vi "SET LPF1.vi"(0 "NMR in":refnum<class "NMR.lvclass">, 5 "CuttOff Freq [MHz]":u8=9 min=1 max=30 step=1, 11 "error in (no error)":errorcluster) -> (4 "NMR out":refnum<class "NMR.lvclass">, 10 "String as ASCII":string, 15 "error out":errorcluster)   [LabVIEW 2011, in "NMR.lvclass"]
uses:
  NMR.lvclass
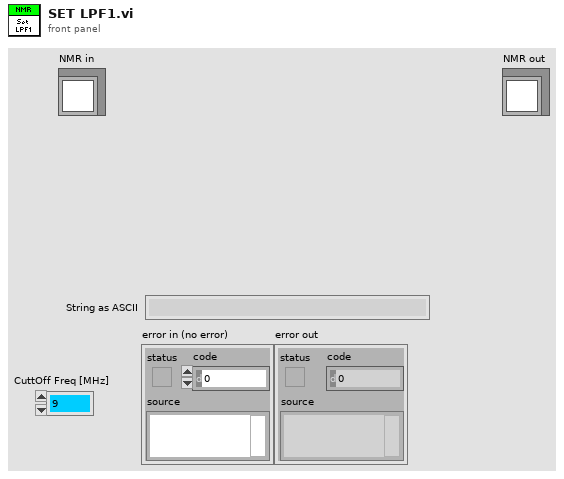
[diagram p1: front panel]
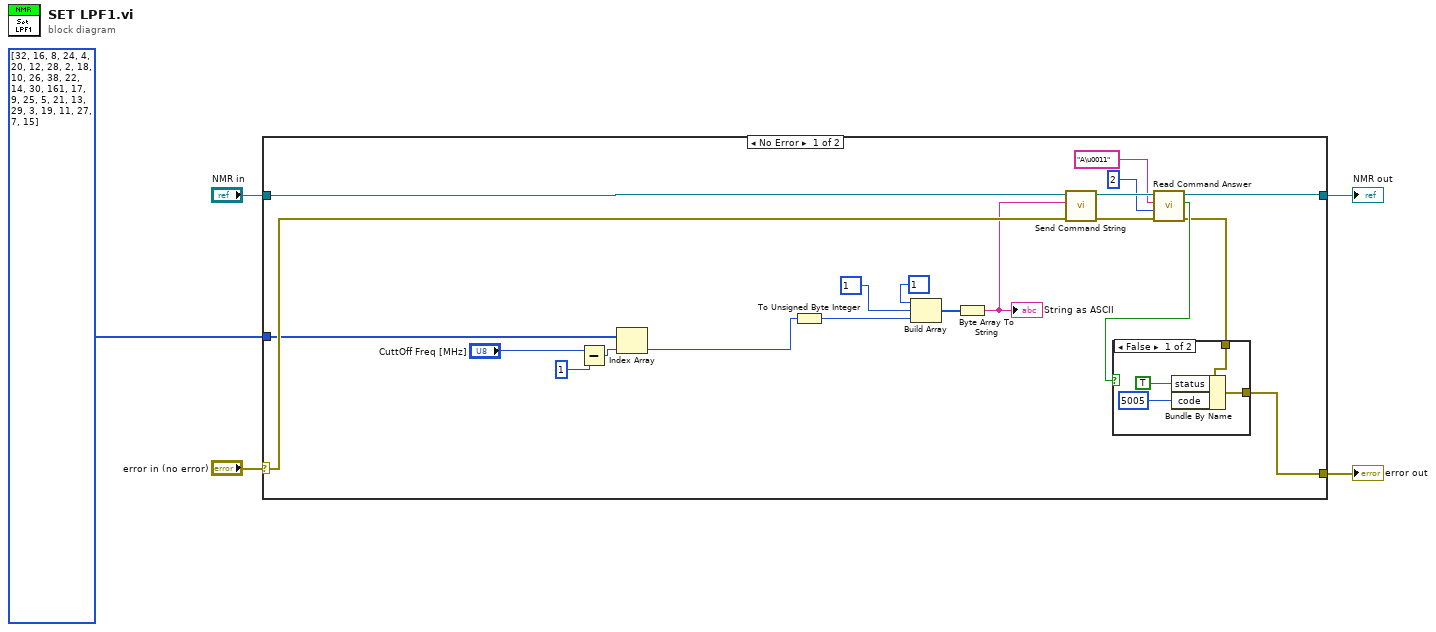
[diagram p0: block diagram]
diagram:
  n1 = case shown="No Error" "error in (no error)" {
    selector: "error in (no error)" -> [w22 w32]
    tunnel: [w12 w32] -> w4
    tunnel: [w23 w31] -> w2
    tunnel: "NMR in" -> [w25 w31]
    tunnel: u8[] [32, 16, 8, 24, 4, 20, 12, 28, 2, 18, 10, 26, 38, 22, 14, 30, 161, 17, 9, 25, 5, 21, 13, 29, 3, 19, 11, 27, 7, 15] -> [w6 _]
    frame No Error {
      n2 = Subtract(x="CuttOff Freq [MHz]", y=u8 1) -> (x-y=w10:u8)
      n3 = Index Array(array=w6, index=w10) -> (element=w7:u8)
      n4 = To Unsigned Byte Integer(number=w7) -> (unsigned 8bit integer=w18:u8)
      n5 = Build Array(u32 1 ("element"), u32 1 ("element"), w18) -> (w20:u32[])
      n6 = Byte Array To String(unsigned byte array=w20) -> (string=w17:string)
      "String as ASCII" <- w17
      n7 = call-dynamic "Send Command String.vi"("error in (no error)"=w22, "Command String"=w17, "NMR in"=w25) -> ("error out"=w21:errorcluster, "NMR out"=w24:refnum<class "NMR.lvclass">)  [unwired: 7 in]
      n8 = call-dynamic "Read Command Answer.vi"("error in (no error)"=w21, "bytes to read"=u32 2 ("Number bytes Read"), "String Seached"="A\u0011" ("search char"), "NMR in"=w24) -> ("error out"=w13:errorcluster, "Expected Answer?"=w14:bool, "NMR out"=w23:refnum<class "NMR.lvclass">)  [unwired: 5 in]
      n9 = case shown="False" w14 {
        tunnel: w13 -> [w27 w30]
        tunnel: [w26 w30] -> w12
        frame False {
          n10 = Bundle By Name(cluster=w27, "status"=TRUE, "code"=5005) -> (w26:errorcluster)
        }
        frame True {
        }
      }
    }
    frame Error {
    }
  }
  "error out" <- w4
  "NMR out" <- w2
